vi "ProductString.vi"(8 "error":errorcluster, 10 "String":string) -> (0 "error  out":errorcluster)   [LabVIEW 2017]
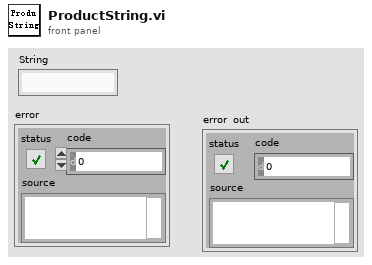
[diagram p1: front panel]
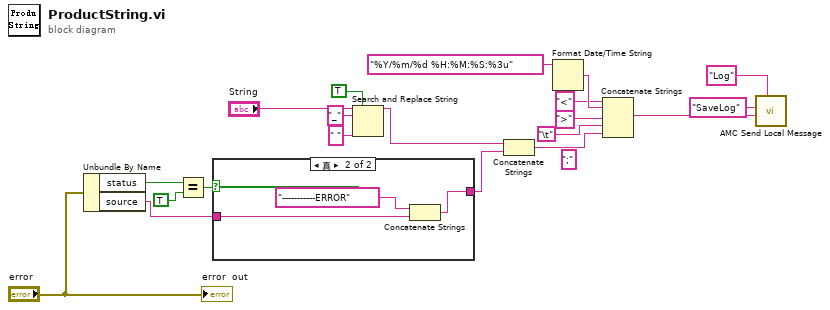
[diagram p0: block diagram]
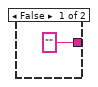
[diagram p2: hidden frame]
diagram:
  (unwired) ";" ("字符串")
  n1 = Unbundle By Name("error") -> ("status"=w20:bool, "source"=w9:string)
  n2 = Equal?(x=w20, y=TRUE) -> (x = y?=w17:bool)
  n3 = case shown="真" w17 {
    tunnel: ["" ("string") w23] -> w18
    tunnel: w9 -> [_ w22]
    frame False {
    }
    frame True {
      n4 = Concatenate Strings("-----------ERROR" ("string"), w22) -> (w23:string)
    }
  }
  n5 = Search and Replace String(replace all?=TRUE ("替换全部？(F)"), input string="String", search string="_" ("搜索字符串"), replace string=" " ("替换字符串(\"\")")) -> (result string=w1:string)  [unwired: 4 in, 3 out]
  n6 = Concatenate Strings(w1, w18) -> (w11:string)
  n7 = Format Date/Time String(time format string (%c)="%Y/%m/%d %H:%M:%S:%3u" ("时间格式字符串(%c)")) -> (date/time string=w16:string)  [unwired: 2 in]
  n8 = Concatenate Strings("<" ("字符串"), w16, ">" ("字符串"), "\t", w11) -> (w10:string)
  n9 = call "AMC Send Local Message.vi"("Process (\"\" - local)"="Log" ("Process (\"\" - local)"), "Message Value"=w10, "Message Name"="SaveLog") -> ()  [unwired: 7 in, 2 out]
  "error  out" <- "error"
